vi "New WS Client.vi"(8 "error in (no error)":errorcluster, 10 "WebSocket Client":refnum<class "WebSocket Client.lvclass">, 11 "Basic WebSocket Manager in":refnum<class "Basic WebSocket Manager.lvclass">) -> (0 "error out":errorcluster)   [LabVIEW 2020, in "HTTP Server.lvlib" / "Basic WebSocket Manager.lvclass"]
uses:
  Basic WebSocket Manager.lvclass
  WebSocket Client/WebSocket Client.lvclass
  <vilib>/Utility/miscctls.llb/LVMapReplaceAction.ctl
  Basic WebSocket Manager.lvclass/Basic WebSocket Manager.ctl
  WebSocket Client/WebSocket Client.lvclass/WebSocket Client.ctl
  lv-http-util/HTTP Utils/Request/Request.lvclass/Request.ctl
  lv-uri/URI/URI/URI.lvclass/URI.ctl
  lv-http-util/HTTP Utils/Request/Get Target URI.vi
  lv-uri/URI/URI/Path String.vi
  lv-http-util/HTTP Utils/Request/Get Client URI.vi
  lv-uri/URI/URI/URI String.vi
  lv-uri/URI/Build URI String.vi
  lv-uri/URI/Build Query String.vi
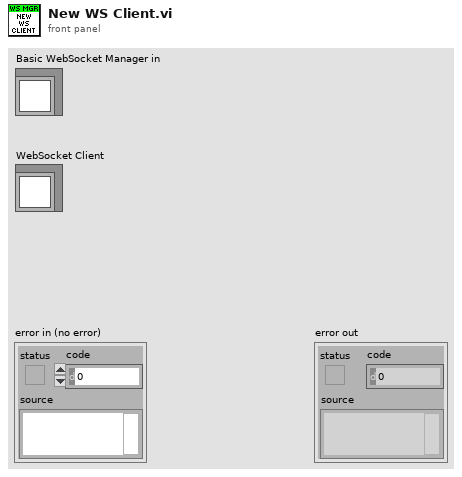
[diagram p1: front panel]
types:
  T1 = typedef "LVMapReplaceAction.ctl" = enum32{"Modify Entry only if found", "Add or Modify Entry", "Delete Entry"}
  T2 = typedef "HTTP Server.lvlib/Basic WebSocket Manager.lvclass/Ref Data.ctl" = cluster{"Clients":map{string, refnum<class "WebSocket Client.lvclass">}}
  T3 = map{string, refnum<class "WebSocket Client.lvclass">}
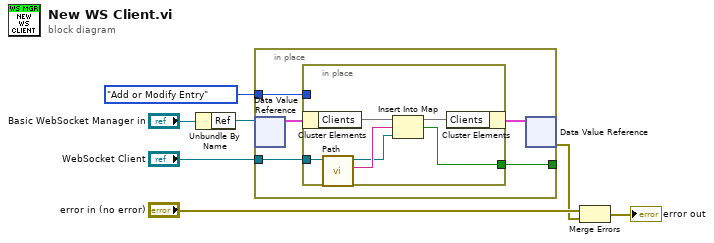
[diagram p0: block diagram]
diagram:
  n1 = Unbundle By Name("Basic WebSocket Manager in") -> ("Ref"=w6:refnum<data-value>)
  n2 = in-place {
    in-place-border: "WebSocket Client" -> [w11]
    in-place-border: LVMapReplaceAction."Add or Modify Entry" ("action") -> [w10]
    in-place-border: [w8] -> _
    n3 = in-place-dvr #1(w6) -> (w12:T2)  [unwired: 1 out]
    n4 = in-place {
      in-place-border: w11 -> [w18]
      in-place-border: w10 -> [_]
      in-place-border: [w13] -> w8
      n5 = in-place-cluster #2(w12) -> ("Clients"=w17:T3)
      n6 = call "Path.vi"("WebSocket Client in"=w18) -> ("Path"=w16:string, "WebSocket Client out"=w15:refnum<class "WebSocket Client.lvclass">)  [unwired: 9 in]
      n7 = Insert Into Map(map in=w17, key=w16, value=w15) -> (map out=w14:T3, key already included?=w13:bool)  [unwired: 1 out]
      n8 = in-place-cluster #2("Clients"=w14) -> (w9:T2)
    }
    n9 = in-place-dvr #1(w9) -> (w1:errorcluster)  [unwired: 1 out]
  }
  n10 = Merge Errors("error in (no error)", w1) -> (→"error out":errorcluster)
